vi "Util_App Application Directory.vi"() -> (3 "Application Directory":path)   [LabVIEW 2016]
doc: "This VI returns the folder containing the current LabVIEW application (top level VI)."
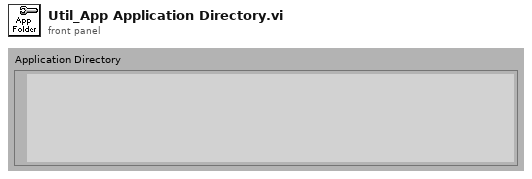
[diagram p1: front panel]
types:
  T1 = enum32{"invalid app kind", "Development System", "Run Time System", "Student Edition", "Embedded LabVIEW", "Evaluation", "Custom"}
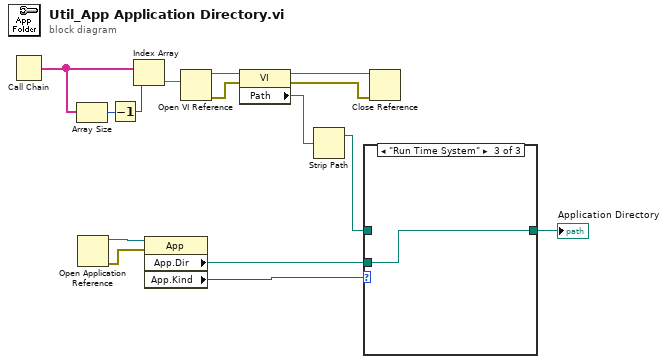
[diagram p0: block diagram]
diagram:
  n1 = Call Chain() -> (call chain=w15:string[])
  n2 = Array Size(array=w15) -> (size(s)=w14:i32)
  n3 = Open Application Reference() -> (0:w5:errorcluster, 3:w6:refnum<vi>)  [unwired: 4 in]
  n4 = Decrement(x=w14) -> (x-1=w13:i32)
  n5 = Index Array(array=w15, index=w13) -> (element=w12:string)
  n6 = property class="App"(reference=w6, error in=w5) -> ("App.Dir"=w1:path, "App.Kind"=w4:T1)  [unwired: 2 out]
  n7 = Open VI Reference(vi path=w12) -> (vi reference=w10:refnum<vi>, error out=w11:errorcluster)  [unwired: 1 in, 4 out]
  n8 = property class="VI"(reference=w10, error in=w11) -> (reference out=w9:refnum<vi>, error out=w8:errorcluster, "Path"=w7:path)
  n9 = Strip Path(path=w7) -> (stripped path=w3:path)  [unwired: 1 out]
  n10 = case shown="\"Run Time System\"" w4 {
    tunnel: [_ w16 w17] -> w2
    tunnel: w3 -> [_ w16 _]
    tunnel: w1 -> [_ _ w17]
    frame Default {
    }
    frame "Development System" {
    }
    frame "Run Time System" {
    }
  }
  "Application Directory" <- w2
  n11 = Close Reference(reference=w9, error in (no error)=w8) -> ()  [unwired: 1 out]
